vi "Basic Control Example.vi"   [LabVIEW 2020]
doc: "This VI is not used in the final software. It is simply a guide to show the starting point of the design methodology as follows:\n- Create a connection to the machine's controller\n- Send some command to perform some action\n- Close the connection to the machine's controller"
uses:
  <instrlib>/Arcus Ethernet Driver 1.0.0/ArcusEthernetComm/classes/Controller/_Controller.lvclass
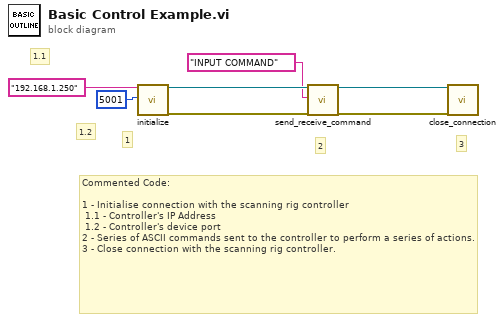
[diagram p0: block diagram]
diagram:
  # "1.2"
  # "1.1"
  # "Commented Code:\n\n1 - Initialise connection with the scanning rig controller \n 1.1 - Controller's IP Address\n 1.2 - Controller's device port\n2 - Series of ASCII commands sent to the controller to perform a series of actions.\n3 - Close connection with the scanning rig controller."
  # "3"
  # "2"
  # "1"
  n1 = call <instrlib>:"initialize.vi"("ip_address (in)"="192.168.1.250", "dev_port(def=5001)"=u16 5001) -> ("reference (out)"=w5:refnum<class "_Controller.lvclass">, "error out"=w3:errorcluster)  [unwired: 16 in]
  n2 = call <instrlib>:"send_receive_command.vi"("reference (in)"=w5, "ASCII Command (in)"="INPUT COMMAND", "error in (no error)"=w3) -> ("reference (out)"=w2:refnum<class "_Controller.lvclass">, "error out"=w1:errorcluster)  [unwired: 12 in, 3 out]
  n3 = call <instrlib>:"close_connection.vi"("reference (in)"=w2, "error in (no error)"=w1) -> ()  [unwired: 16 in, 2 out]
